vi "Joystick-Manual.vi"() -> ()   [LabVIEW 2012]
uses:
  <vilib>/Utility/inputDevices.llb/closeJoystick.vi
  <vilib>/Utility/inputDevices.llb/joystickAcquire.vi
panel:
  in  "Communication":bool caption="Stop (F)"
  in  "Remote UDP Port":u16=61557
  in  "Local Port":u16=61556
  in  "Remote Host":string="localhost"
  in  "broadcast":bool
  out "rot-":bool
  out "rot+":bool
  out "y-":bool
  out "y+":bool
  out "x-":bool
  out "x+":bool
  out "Float":bool
  in  "stop":bool
  out "axis info":T1
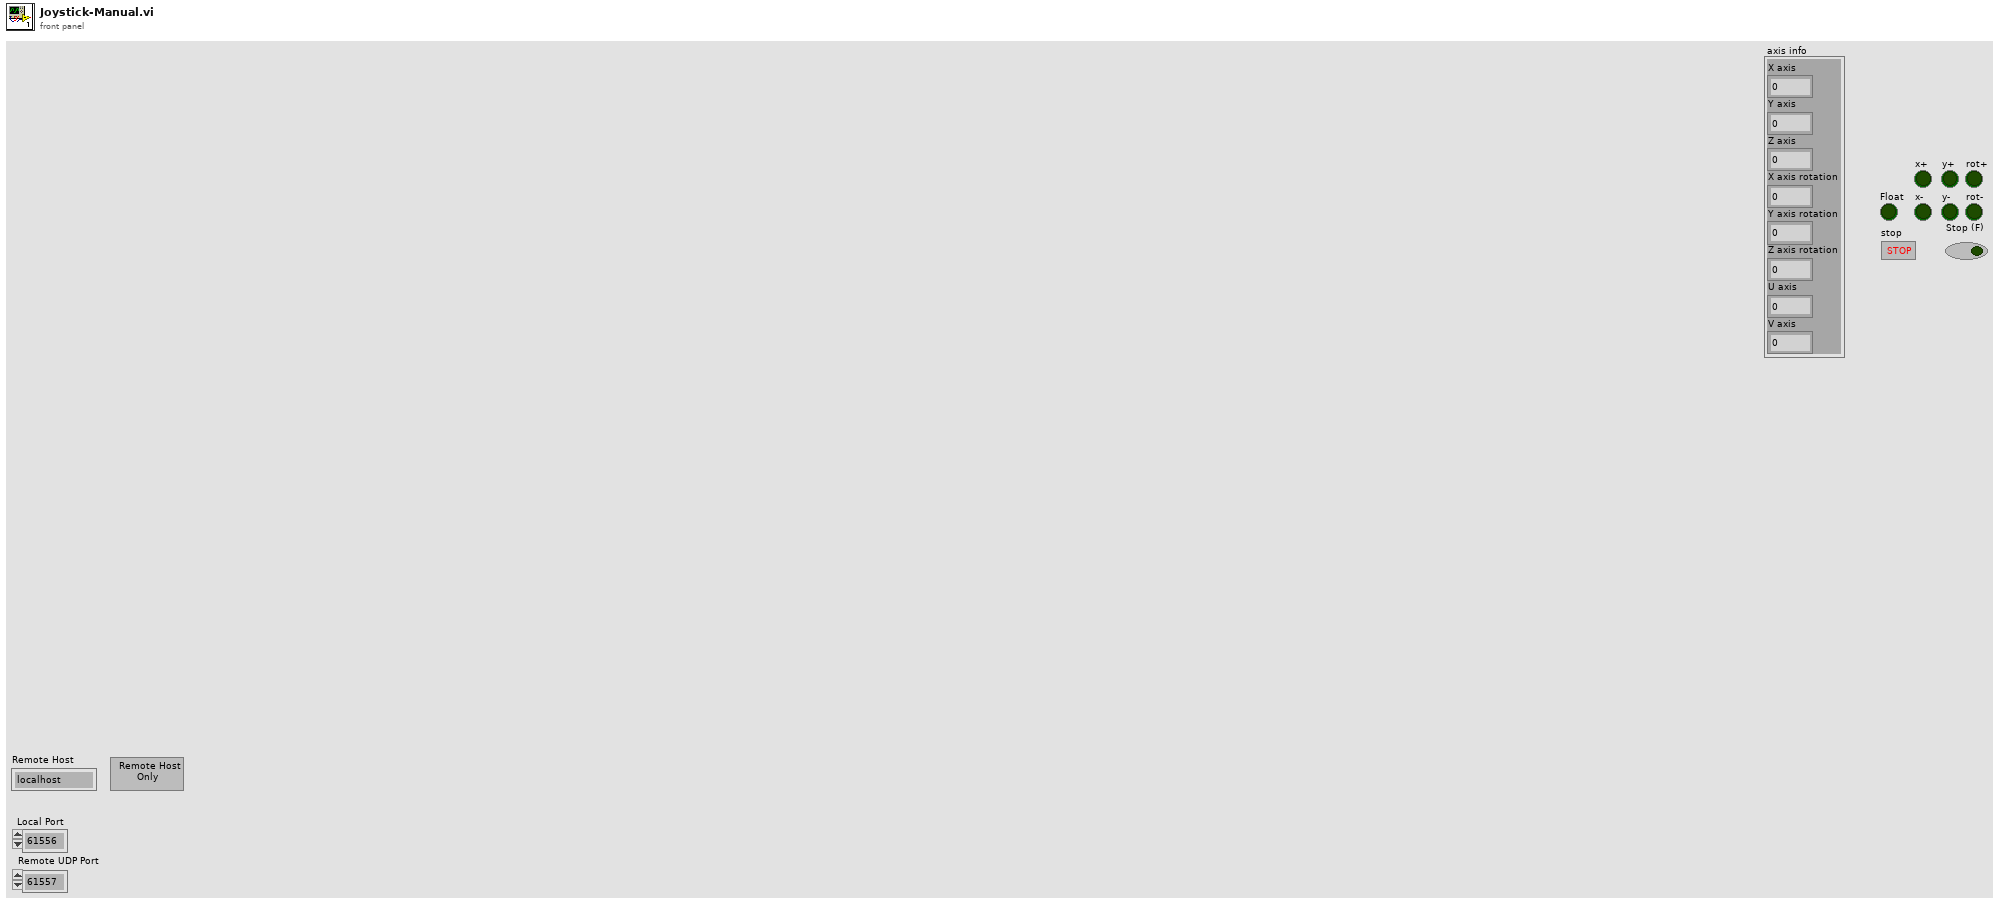
[diagram p1: front panel]
types:
  T1 = cluster{"X axis":i32, "Y axis":i32, "Z axis":i32, "X axis rotation":i32, "Y axis rotation":i32, "Z axis rotation":i32, "U axis":i32, "V axis":i32}
  T2 = cluster{"x+":bool, "x-":bool, "y+":bool, "y-":bool, "rot+":bool, "rot-":bool, "Float":bool}
  T3 = cluster{"button 1":bool, "button 2":bool, "button 3":bool, "button 4":bool, "button 5":bool, "button 6":bool, "button 7":bool, "button 8":bool, "button 9":bool, "button 10":bool, "button 11":bool, "button 12":bool, "button 13":bool, "button 14":bool, "button 15":bool, "button 16":bool, "button 17":bool, "button 18":bool, "button 19":bool, "button 20":bool, "button 21":bool, "button 22":bool, "button 23":bool, "button 24":bool, "button 25":bool, "button 26":bool, "button 27":bool, "button 28":bool, "button 29":bool, "button 30":bool, "button 31":bool, "button 32":bool}
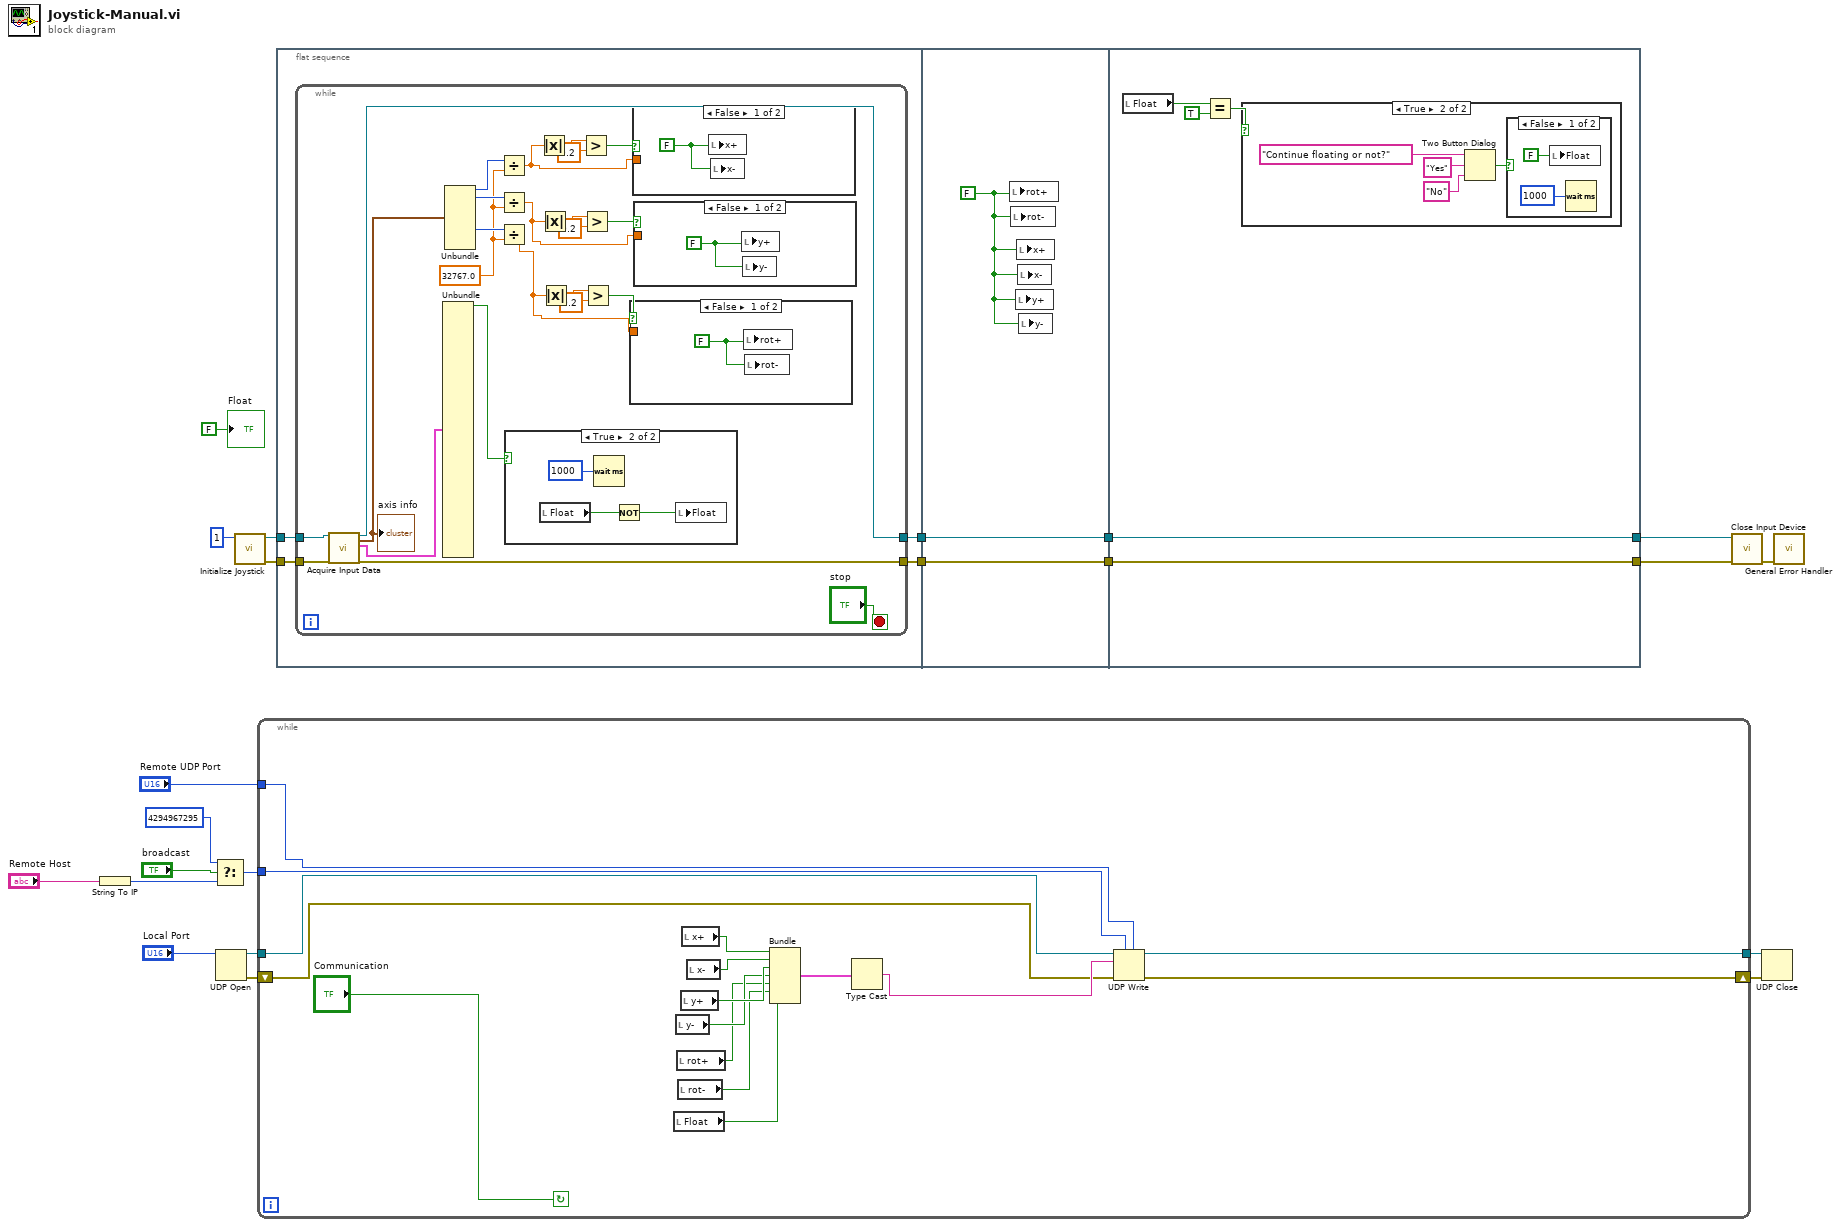
[diagram p0: block diagram]
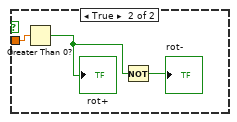
[diagram p2: hidden frame]
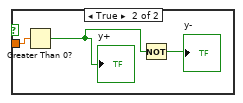
[diagram p3: hidden frame]
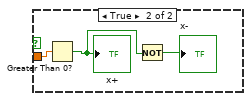
[diagram p4: hidden frame]
diagram:
  n1 = String To IP(1:"Remote Host") -> (0:w8:u32)
  n2 = Select(t=u32 4294967295, s="broadcast", f=w8) -> (s? t:f=w5:u32)
  n3 = UDP Open(11:"Local Port") -> (port=w4:refnum<k16>, 0:w3:errorcluster)  [unwired: 1 in, 4 out]
  n4 = call <vilib>:"Initialize Joystick.vi"("device index"=1) -> ("error out"=w17:errorcluster, "device ID"=w16:refnum<k1>)  [unwired: 9 in]
  n5 = while {
    tunnel: "Remote UDP Port" -> [w38]
    tunnel: w5 -> [w37]
    tunnel: w4 -> [w23]
    tunnel: [w35] -> w2
    shift-right: [w34] -> w1
    shift-left: w3 -> [w24]
    stop <- "Communication" continue-if-true
    n6 = local read "Float"() -> (w27:bool)
    n7 = local read "y-"() -> (w30:bool)
    n8 = local read "rot+"() -> (w29:bool)
    n9 = local read "rot-"() -> (w28:bool)
    n10 = local read "y+"() -> (w31:bool)
    n11 = local read "x+"() -> (w33:bool)
    n12 = local read "x-"() -> (w32:bool)
    n13 = Bundle("x+"=w33, "x-"=w32, "y+"=w31, "y-"=w30, "rot+"=w29, "rot-"=w28, "Float"=w27) -> (w26:T2)  [unwired: 1 in]
    n14 = Type Cast(x=w26) -> (*(type *) &x=w25:string)  [unwired: 1 in]
    n15 = UDP Write(address=w37, port or service name=w38, connection ID=w23, data in=w25, 8:w24) -> (error out=w34:errorcluster, 3:w35:refnum<k16>)  [unwired: 1 out]
  }
  n16 = flat-sequence {
    tunnel: w17 -> [w40]
    tunnel: w16 -> [w39]
    tunnel: [w42] -> w15
    tunnel: [w41] -> w13
    tunnel: w15 -> [w84]
    tunnel: [w84] -> w14
    tunnel: w13 -> [w83]
    tunnel: [w83] -> w12
    tunnel: [w88] -> w20
    tunnel: [w89] -> w21
    tunnel: w14 -> [w89]
    tunnel: w12 -> [w88]
    frame #0 {
      n17 = while {
        tunnel: [w60] -> w42
        tunnel: [w59] -> w41
        tunnel: w39 -> [w58]
        tunnel: w40 -> [w57]
        stop <- "stop" stop-if-true
        w62 = 32767.0 ("y")
        n18 = call-poly <vilib>:"Acquire Input Data.vi"("device ID"=w58, "error in (no error)"=w57) -> ("device ID"=w60:refnum<k1>, "axis info"=w66:T1, "button info"=w61:T3, "error out"=w59:errorcluster)  [unwired: 13 in, 1 out]
        "axis info" <- w66
        n19 = Unbundle(w61) -> ("button 1"=w55:bool)  [unwired: 31 out]
        n20 = Unbundle(w66) -> ("X axis"=w65:i32, "Y axis"=w64:i32, "Z axis rotation"=w63:i32)  [unwired: 5 out]
        n21 = Divide(x=w65, y=w62) -> (x/y=w51:dbl)
        n22 = Divide(x=w64, y=w62) -> (x/y=w47:dbl)
        n23 = Divide(x=w63, y=w62) -> (x/y=w43:dbl)
        n24 = case shown="True" w55 {
          frame False {
          }
          frame True {
            n25 = local read "Float"() -> (w81:bool)
            n26 = Wait (ms)(milliseconds to wait=u32 1000) -> ()  [unwired: 1 out]
            n27 = Not(x=w81) -> (.not. x?=w80:bool)
            n28 = local write "Float"(w80) -> ()
          }
        }
        n29 = Absolute Value(x=w51) -> (abs(x)=w54:dbl)
        n30 = Absolute Value(x=w47) -> (abs(x)=w50:dbl)
        n31 = Absolute Value(x=w43) -> (abs(x)=w46:dbl)
        n32 = Greater?(x=w54, y=0.2) -> (0:w52:bool)
        n33 = Greater?(x=w50, y=0.2) -> (0:w48:bool)
        n34 = Greater?(x=w46, y=0.2) -> (0:w44:bool)
        n35 = case shown="False" w44 {
          tunnel: w43 -> [_ w70]
          frame False {
            w67 = FALSE
            n36 = local write "rot+"(w67) -> ()
            n37 = local write "rot-"(w67) -> ()
          }
          frame True {
            n38 = Greater Than 0?(x=w70) -> (x > 0?=w69:bool)
            "rot+" <- w69
            n39 = Not(x=w69) -> (.not. x?=→"rot-":bool)
          }
        }
        n40 = case shown="False" w52 {
          tunnel: w51 -> [_ w78]
          frame False {
            w75 = FALSE
            n41 = local write "x+"(w75) -> ()
            n42 = local write "x-"(w75) -> ()
          }
          frame True {
            n43 = Greater Than 0?(x=w78) -> (x > 0?=w77:bool)
            "x+" <- w77
            n44 = Not(x=w77) -> (.not. x?=→"x-":bool)
          }
        }
        n45 = case shown="False" w48 {
          tunnel: w47 -> [_ w74]
          frame False {
            w71 = FALSE
            n46 = local write "y+"(w71) -> ()
            n47 = local write "y-"(w71) -> ()
          }
          frame True {
            n48 = Greater Than 0?(x=w74) -> (x > 0?=w73:bool)
            "y+" <- w73
            n49 = Not(x=w73) -> (.not. x?=→"y-":bool)
          }
        }
      }
    }
    frame #1 {
      w82 = FALSE
      n50 = local write "rot+"(w82) -> ()
      n51 = local write "rot-"(w82) -> ()
      n52 = local write "y+"(w82) -> ()
      n53 = local write "x+"(w82) -> ()
      n54 = local write "x-"(w82) -> ()
      n55 = local write "y-"(w82) -> ()
    }
    frame #2 {
      n56 = local read "Float"() -> (w87:bool)
      n57 = Equal?(x=w87, y=TRUE) -> (x = y?=w85:bool)
      n58 = case shown="True" w85 {
        frame False {
        }
        frame True {
          n59 = Two Button Dialog(message="Continue floating or not?", 1:"No" ("F button name (\"Cancel\")"), 2:"Yes" ("T button name (\"OK\")")) -> (T button?=w90:bool)
          n60 = case shown="False" w90 {
            frame False {
              n61 = local write "Float"(FALSE) -> ()
              n62 = Wait (ms)(milliseconds to wait=u32 1000) -> ()  [unwired: 1 out]
            }
            frame True {
            }
          }
        }
      }
    }
  }
  n63 = call-poly <vilib>:"Close Input Device.vi"("error in (no error)"=w20, "device ID"=w21) -> ("error out"=w19:errorcluster)  [unwired: 8 in]
  n64 = UDP Close(connection ID=w2, 8:w1) -> ()  [unwired: 2 out]
  n65 = call <vilib>:"General Error Handler.vi"("error in (no error)"=w19) -> ()  [unwired: 1 in, 14 out]
  "Float" <- FALSE
